vi "Initialization VI.vi"(8 "error in (no error)":errorcluster, 10 "Custom XML":string, 11 "Device Item Ref in":T1 format="%.0x") -> (0 "error out":errorcluster, 3 "Device Item Ref out":T1 format="%.0x")   [LabVIEW 2019, in "RMXVisaControl System Explorer.lvlib"]
uses:
  RMXVisaControl System Explorer.lvlib
  <vilib>/NI VeriStand/Custom Device API/Custom Device Item Ref.ctl
  <vilib>/NI VeriStand/Custom Device API/Custom Device Channel.ctl
  <vilib>/NI VeriStand/Custom Device API/Custom Device Channel Type.ctl
  Shared/Constants.vi
  <vilib>/NI VeriStand/Custom Device API/Custom Device API.lvlib
  Shared/RMXVisaControl Shared.lvlib
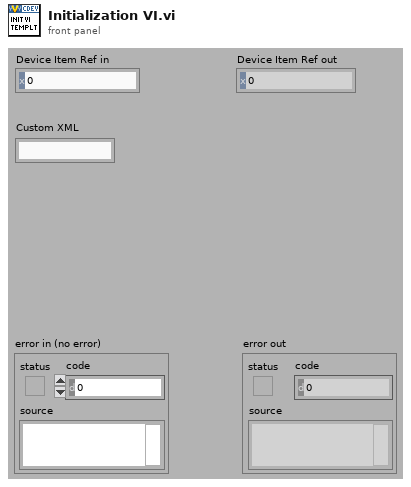
[diagram p1: front panel]
types:
  T1 = typedef "Custom Device API.lvlib/Custom Device Item Ref.ctl" = u64
  T2 = typedef "Custom Device API.lvlib/Custom Device Channel.ctl" = cluster{"Type":T3, "Units":string, "Default Value":dbl, "Faultable":bool, "Scalable":bool}
  T3 = typedef "Custom Device API.lvlib/Custom Device Channel Type.ctl" = enum16{"Input", "Output"}
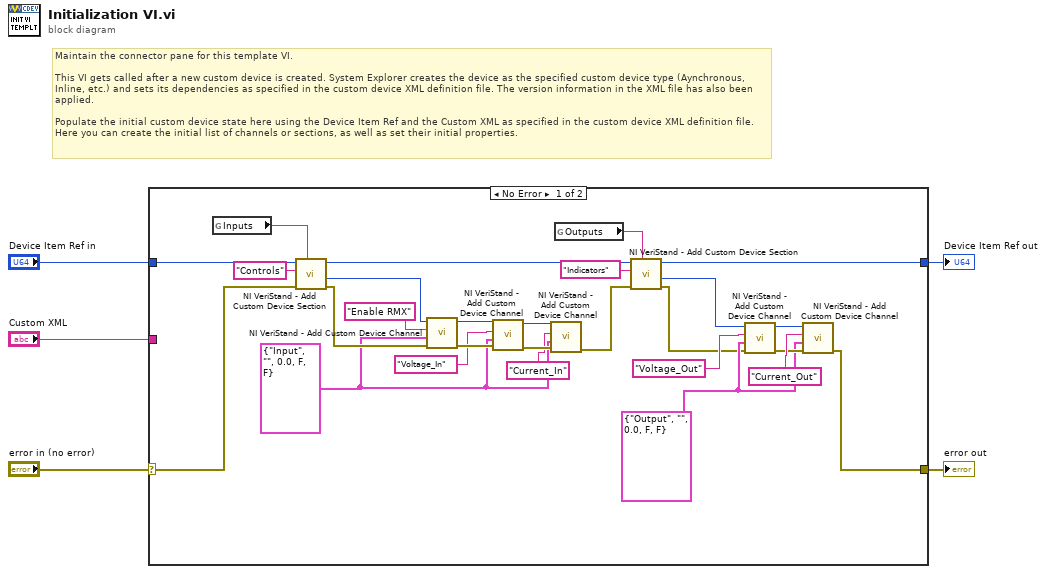
[diagram p0: block diagram]
diagram:
  # "Maintain the connector pane for this template VI.\n\nThis VI gets called after a new custom device is created. System Explorer creates the device as the specified custom device type (Aynchronous, Inline, etc.) and sets its dependencies as specified in the custom device XML definition file. The version information in the XML file has also been applied.\n\nPopulate the initial custom device state here using the Device Item Ref and the Custom XML as specified in the custom device XML definition file. Here you can create the initial list of channels or sections, as well as set their initial properties."
  n1 = case shown="No Error" "error in (no error)" {
    selector: "error in (no error)" -> [w10 w34]
    tunnel: [w9 w34] -> w5
    tunnel: [w31 w33] -> w3
    tunnel: "Device Item Ref in" -> [w32 w33]
    tunnel: "Custom XML" -> [_ _]
    frame No Error {
      w14 = T2 {"Type"=enum."Output", "Units"="", "Default Value"=0.0, "Faultable"=FALSE, "Scalable"=FALSE} ("Channel")
      w18 = T2 {"Type"=enum."Input", "Units"="", "Default Value"=0.0, "Faultable"=FALSE, "Scalable"=FALSE} ("Channel")
      n2 = global read "Constants.vi" "Inputs"() -> (w7:string)
      n3 = call <vilib>:"NI VeriStand - Add Custom Device Section.vi"("GUID (Default Section)"=w7, "error in (no error)"=w10, "Section Name"="Controls", "Parent Ref in"=w32) -> ("error out"=w23:errorcluster, "Section Ptr"=w27:T1, "Parent Ref out"=w28:T1)  [unwired: 4 in, 1 out]
      n4 = call <vilib>:"NI VeriStand - Add Custom Device Channel.vi"("error in (no error)"=w23, "Channel"=w18, "Channel Name"="Enable RMX", "Parent Ref in"=w27) -> ("error out"=w24:errorcluster, "Parent Ref out"=w25:T1)  [unwired: 4 in, 2 out]
      n5 = call <vilib>:"NI VeriStand - Add Custom Device Channel.vi"("error in (no error)"=w24, "Channel"=w18, "Channel Name"="Voltage_In", "Parent Ref in"=w25) -> ("error out"=w21:errorcluster, "Parent Ref out"=w20:T1)  [unwired: 4 in, 2 out]
      n6 = call <vilib>:"NI VeriStand - Add Custom Device Channel.vi"("error in (no error)"=w21, "Channel"=w18, "Channel Name"="Current_In", "Parent Ref in"=w20) -> ("error out"=w13:errorcluster)  [unwired: 4 in, 3 out]
      n7 = global read "Constants.vi" "Outputs"() -> (w6:string)
      n8 = call <vilib>:"NI VeriStand - Add Custom Device Section.vi"("GUID (Default Section)"=w6, "error in (no error)"=w13, "Section Name"="Indicators", "Parent Ref in"=w28) -> ("error out"=w12:errorcluster, "Section Ptr"=w11:T1, "Parent Ref out"=w31:T1)  [unwired: 4 in, 1 out]
      n9 = call <vilib>:"NI VeriStand - Add Custom Device Channel.vi"("error in (no error)"=w12, "Channel"=w14, "Channel Name"="Voltage_Out", "Parent Ref in"=w11) -> ("error out"=w16:errorcluster, "Parent Ref out"=w8:T1)  [unwired: 4 in, 2 out]
      n10 = call <vilib>:"NI VeriStand - Add Custom Device Channel.vi"("error in (no error)"=w16, "Channel"=w14, "Channel Name"="Current_Out", "Parent Ref in"=w8) -> ("error out"=w9:errorcluster)  [unwired: 4 in, 3 out]
    }
    frame Error {
    }
  }
  "error out" <- w5
  "Device Item Ref out" <- w3
